vi "Test - Bird to Coords.vi"() -> ()   [LabVIEW 2013]
panel:
  out "Tube":i16[][](graph)
  out "Bird":i16[][](graph)
  out "Image Pixels (U32)":u32[][](graph)
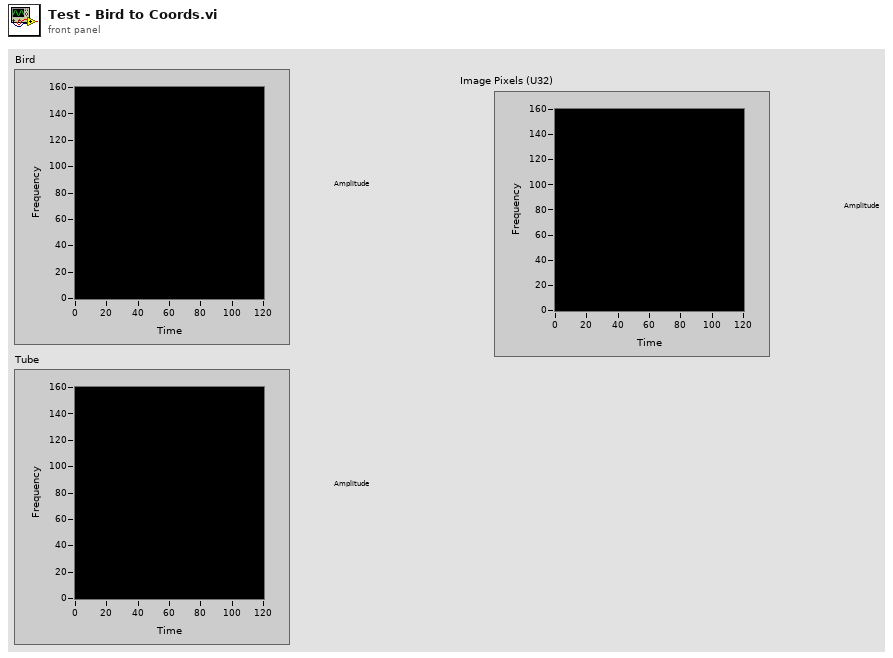
[diagram p1: front panel]
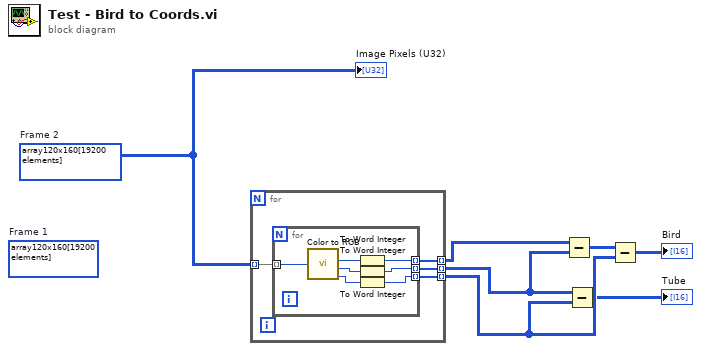
[diagram p0: block diagram]
diagram:
  w1 = u32[][] array120x160[19200 elements]  # Frame 2
  (unwired) u32[][] array120x160[19200 elements]  # Frame 1
  n1 = for {
    tunnel: w1 -> [w11] mode=indexing
    tunnel: [w10] -> w7 mode=indexing
    tunnel: [w9] -> w4 mode=indexing
    tunnel: [w8] -> w3 mode=indexing
    n2 = for {
      tunnel: w11 -> [w18] mode=indexing
      tunnel: [w16] -> w10 mode=indexing
      tunnel: [w13] -> w9 mode=indexing
      tunnel: [w12] -> w8 mode=indexing
      n3 = call <vilib>:"Color to RGB.vi"("Color"=w18) -> ("R"=w17:u8, "G"=w14:u8, "B"=w15:u8)  [unwired: 1 out]
      n4 = To Word Integer(number=w17) -> (16bit integer=w16:i16)
      n5 = To Word Integer(number=w14) -> (16bit integer=w13:i16)
      n6 = To Word Integer(number=w15) -> (16bit integer=w12:i16)
    }
  }
  n7 = Subtract(x=w7, y=w4) -> (x-y=w6:i16[][])
  n8 = Subtract(x=w4, y=w3) -> (x-y=→"Tube":i16[][])
  n9 = Subtract(x=w6, y=w3) -> (x-y=→"Bird":i16[][])
  "Image Pixels (U32)" <- w1
